vi "DHE_ReadTP.vi"(4 "Database RefNum in":T1, 6 "phys. unit":string, 7 "switches":string[](array[string]), 8 "error in (no error)":errorcluster, 9 "index in":i32, 10 "TP In":T2={"name"="", "type"="", "R_algor"=[], "board"="", "memory"="", "address"=0, "value"="", "Limits"={"upper"=0.0, "Lower"=0.0, "InRange"=FALSE, "nominal"=0.0}, "unit"="", "params"="", "permissions"="", "W_algor"=[], "description"="", "err_count"=0, "max_err"=3, "read"=FALSE, "lowrej"=0.0, "hirej"=0.0, "expupd"=FALSE} {"Limits"."nominal" format="%.2f"; "Limits"."Lower" format="%.2f"; "Limits"."upper" format="%.2f"}, 11 "refnum":i32) -> (0 "error out":errorcluster, 1 "In Range?":bool, 2 "response":string, 3 "refnum out":i32)   [LabVIEW 2016]
uses:
  DHE_TP.ctl
  DHE_TPLimits.ctl
  DBSHAND/private/vis/DatabaseHand_RefNum.ctl
  DHE_TP_action.ctl
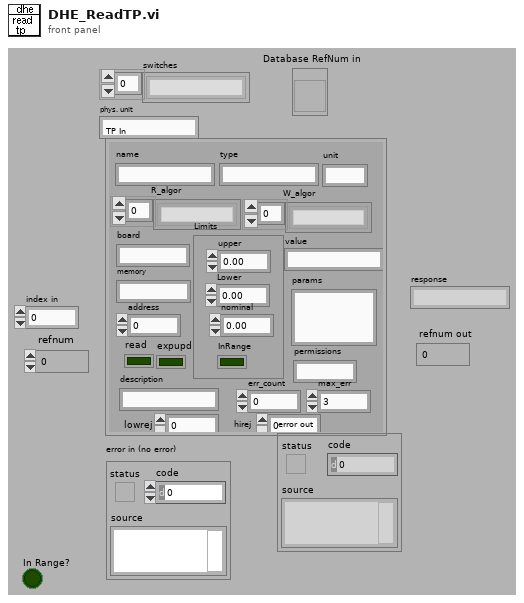
[diagram p1: front panel]
types:
  T1 = typedef "DatabaseHand_RefNum.ctl" = refnum<vi>
  T2 = typedef "DHE_TP.ctl" = cluster{"name":string, "type":string, "R_algor":string[], "board":string, "memory":string, "address":i32, "value":string, "Limits":T3, "unit":string, "params":string, "permissions":string, "W_algor":string[], "description":string, "err_count":i32, "max_err":i32, "read":bool, "lowrej":dbl, "hirej":dbl, "expupd":bool}
  T3 = typedef "DHE_TPLimits.ctl" = cluster{"upper":dbl, "Lower":dbl, "InRange":bool, "nominal":dbl}
  T4 = enum16{"Idle", "Exposing", "Paused", "AbortExp", "Reading", "AbortRead", "FinishedReading", "Resetting", "Reducing", "Initializing"}
  T5 = typedef "DHE_TP_action.ctl" = enum16{"READ FROM FILE", "GET ALL", "FIND BY NAME", "FIND BY TYPE", "SET VALUE", "CLEAN", "CHANGE", "GET EXPUPDATE"}
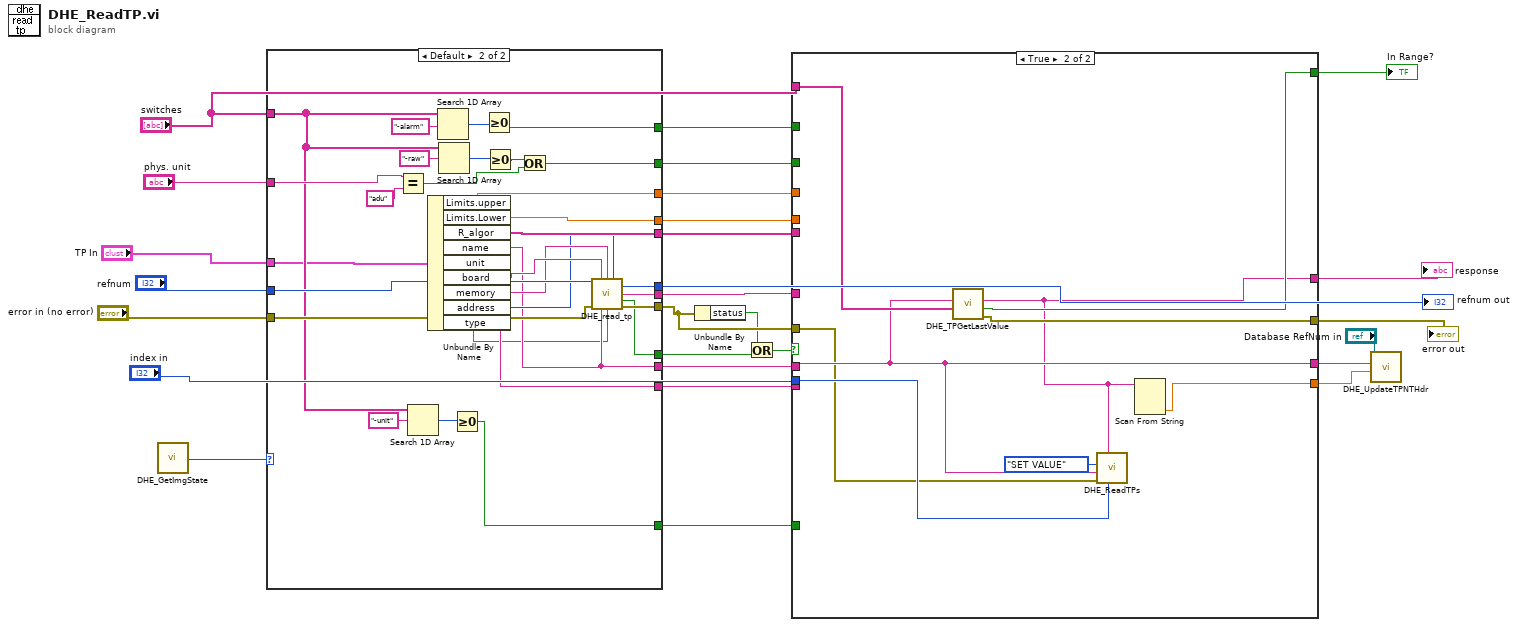
[diagram p0: block diagram]
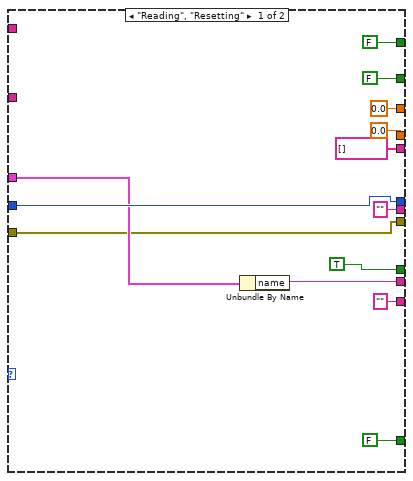
[diagram p2: hidden frame]
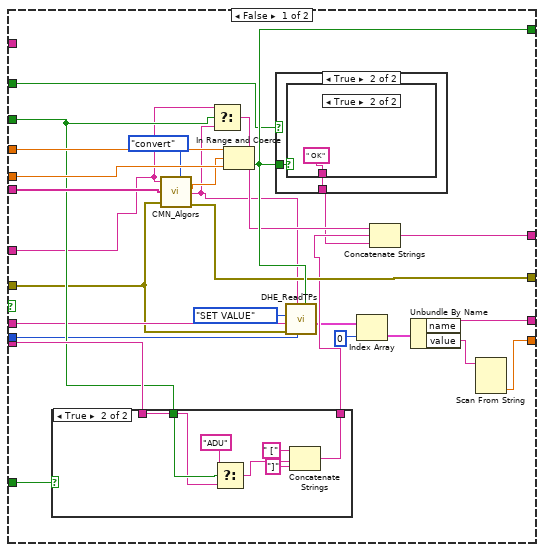
[diagram p3: hidden frame]
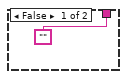
[diagram p4: hidden frame]
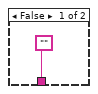
[diagram p5: hidden frame]
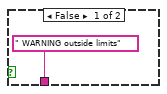
[diagram p6: hidden frame]
diagram:
  n1 = call "DHE_GetImgState.vi"() -> ("DHE_ImgState"=w5:T4)  [unwired: 9 out]
  n2 = case shown="Default" w5 {
    tunnel: [0.0 ("upper") w70] -> w27
    tunnel: [0.0 ("Lower") w69] -> w26
    tunnel: [string[] [] ("R_algor") w66] -> w23
    tunnel: [FALSE w63] -> w21
    tunnel: [FALSE w60] -> w20
    tunnel: ["" ("unit") w59] -> w19
    tunnel: [FALSE w57] -> w18
    tunnel: "phys. unit" -> [_ w54]
    tunnel: "refnum" -> [w37 w53]
    tunnel: "error in (no error)" -> [w28 w52]
    tunnel: [w37 w51] -> w12
    tunnel: ["" ("return value") w47] -> w11
    tunnel: [w30 w46] -> w10
    tunnel: [w28 w44] -> w4
    tunnel: "switches" -> [_ w43]
    tunnel: "TP In" -> [w31 w42]
    tunnel: [TRUE ("y") w41] -> w1
    frame "Reading", "Resetting" {
      n3 = Unbundle By Name(w31) -> ("name"=w30:string)
    }
    frame Default {
      n4 = Equal?(x=w54, y="adu") -> (x = y?=w55:bool)
      n5 = Search 1D Array(1D array=w43, element="-unit") -> (index of element=w61:i32)  [unwired: 1 out]
      n6 = Unbundle By Name(w42) -> ("Limits.upper"=w70:dbl, "Limits.Lower"=w69:dbl, "R_algor"=w66:string[], "name"=w46:string, "unit"=w59:string, "board"=w50:string, "memory"=w49:string, "address"=w48:i32, "type"=w45:string)
      n7 = Search 1D Array(1D array=w43, element="-alarm") -> (index of element=w64:i32)  [unwired: 1 out]
      n8 = Search 1D Array(1D array=w43, element="-raw") -> (index of element=w67:i32)  [unwired: 1 out]
      n9 = Greater Or Equal To 0?(x=w61) -> (x >= 0?=w60:bool)
      n10 = Greater Or Equal To 0?(x=w64) -> (x >= 0?=w63:bool)
      n11 = Greater Or Equal To 0?(x=w67) -> (x >= 0?=w58:bool)
      n12 = Or(x=w58, y=w55) -> (x .or. y?=w57:bool)
      n13 = call "DHE_read_tp.vi"("fd"=w53, "board"=w50, "memory"=w49, "address"=w48, "error in (no error)"=w52, "name"=w46, "type"=w45) -> ("fd out"=w51:i32, "return value"=w47:string, "busy"=w41:bool, "error out"=w44:errorcluster)  [unwired: 5 out]
    }
  }
  "refnum out" <- w12
  n14 = Unbundle By Name(w4) -> ("status"=w3:bool)
  n15 = Or(x=w3, y=w1) -> (x .or. y?=w2:bool)
  n16 = case shown="True" w2 {
    tunnel: w27 -> [w97 _]
    tunnel: w26 -> [w96 _]
    tunnel: [w95 w113] -> w25
    tunnel: [w93 w118] -> w24
    tunnel: w23 -> [w91 _]
    tunnel: [w90 w115] -> w22
    tunnel: w21 -> [w88 _]
    tunnel: w20 -> [w87 _]
    tunnel: w19 -> [w86 _]
    tunnel: w18 -> [w85 _]
    tunnel: "index in" -> [w82 w116]
    tunnel: w11 -> [w79 _]
    tunnel: w10 -> [w78 w117]
    tunnel: [w76 w117] -> w9
    tunnel: [w72 w112] -> w8
    tunnel: "switches" -> [_ w119]
    tunnel: w4 -> [w75 w114]
    frame False {
      n17 = case shown="True" w87 {
        tunnel: w86 -> [_ w102]
        tunnel: w85 -> [_ w103]
        tunnel: ["" w99] -> w84
        frame False {
        }
        frame True {
          n18 = Select(t="ADU", s=w103, f=w102) -> (s? t:f=w100:string)
          n19 = Concatenate Strings(" [" ("string"), w100, "]" ("string")) -> (w99:string)
        }
      }
      n20 = call "CMN_Algors.vi"("ValueIn"=w79, "algors"=w91, "error in (no error)"=w75, "action"=enum16{"convert", "read from file", "get"}."convert") -> ("Value out"=w94:sgl, "string value"=w74:string, "error out"=w90:errorcluster)  [unwired: 1 in, 3 out]
      n21 = Select(t=w79, s=w85, f=w74) -> (s? t:f=w92:string)
      n22 = In Range and Coerce(upper limit=w97, x=w94, lower limit=w96) -> (In Range?=w93:bool)  [unwired: 1 out]
      n23 = case shown="True" w88 {
        tunnel: ["" w108] -> w83
        tunnel: w93 -> [_ w107]
        frame False {
        }
        frame True {
          n24 = case shown="True" w107 {
            tunnel: [" WARNING outside limits" " OK"] -> w108
            frame False {
            }
            frame True {
            }
          }
        }
      }
      n25 = call "DHE_ReadTPs.vi"("inRange"=w93, "index in"=w82, "value"=w74, "error in (no error)"=w75, "argument"=w78, "action"=DHE_TP_action."SET VALUE") -> ("TPs"=w81:T2[])  [unwired: 1 in, 4 out]
      n26 = Index Array(array=w81, index=0) -> (element=w77:T2)
      n27 = Concatenate Strings(w92, w84, w83) -> (w95:string)
      n28 = Unbundle By Name(w77) -> ("name"=w76:string, "value"=w73:string)
      n29 = Scan From String(input string=w73) -> (output 1=w72:dbl)  [unwired: 3 in, 4 out]
    }
    frame True {
      n30 = call "DHE_TPGetLastValue.vi"("swhitches"=w119, "name"=w117) -> ("error IO"=w115:errorcluster, "Limits.InRange"=w118:bool, "value"=w113:string)  [unwired: 1 in, 6 out]
      n31 = call "DHE_ReadTPs.vi"("index in"=w116, "value"=w113, "error in (no error)"=w114, "argument"=w117, "action"=DHE_TP_action."SET VALUE") -> ()  [unwired: 2 in, 5 out]
      n32 = Scan From String(input string=w113) -> (output 1=w112:dbl)  [unwired: 3 in, 4 out]
    }
  }
  "response" <- w25
  "error out" <- w22
  "In Range?" <- w24
  n33 = call "DHE_UpdateTPNTHdr.vi"("TP value"=w8, "TP name"=w9, "Database RefNum in"="Database RefNum in") -> ()  [unwired: 1 in, 8 out]
